vi "compileRfOutputList.vi"(8 "error in (no error)":errorcluster, 11 "ScriptListCompiler in":refnum<class "ScriptListCompiler.lvclass">) -> (0 "error out":errorcluster, 3 "ScriptListCompiler out":refnum<class "ScriptListCompiler.lvclass">)   [LabVIEW 2009, in "Compiler.lvlib" / "ScriptListCompiler.lvclass"]
doc: "Compiles the Analog ScriptList.\n i) Applies the calibration.\n ii) Split Analog List by device.\n iii) Produces digital trigger pulses (for each device) making Digital ScriptLists."
uses:
  ScriptListCompiler.lvclass
  ScriptListCompiler.lvclass/ScriptListCompiler.ctl
  Scripting/ScriptingEvent/ScriptEventList/ScriptEventList.lvclass
  DatabaseHelpers/DbConnection/DeviceDataBase/deviceDataBase.lvclass
  DatabaseHelpers/Database Objects/DeviceArray/DeviceArray.lvclass
  DatabaseHelpers/Database Objects/device/device.lvclass
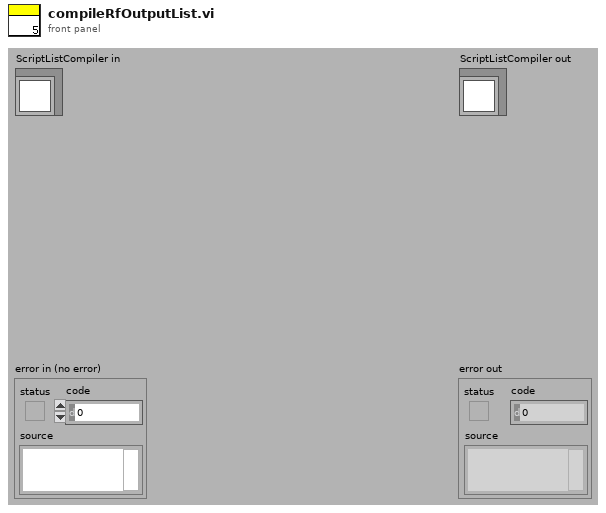
[diagram p1: front panel]
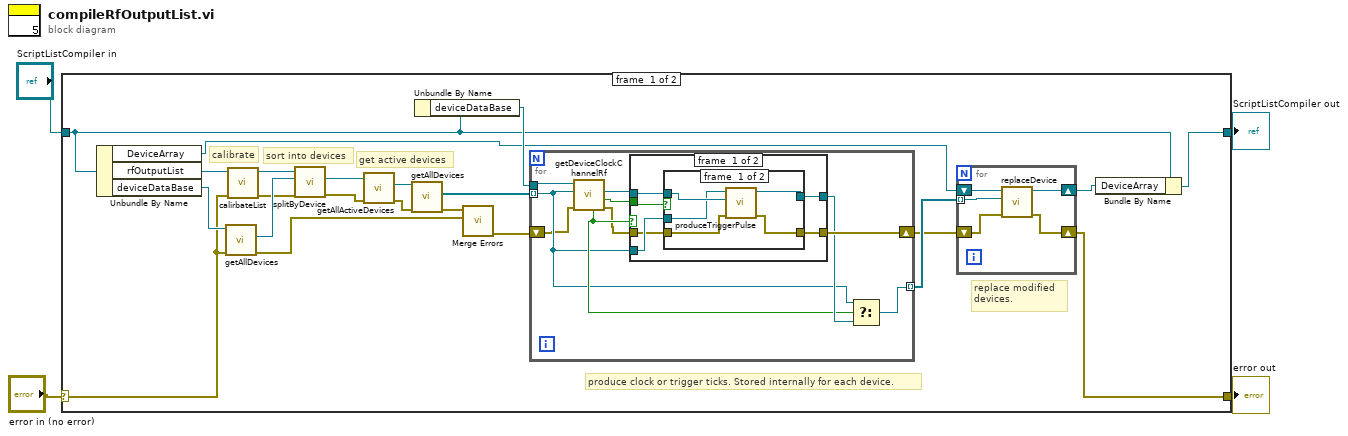
[diagram p0: block diagram]
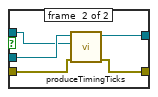
[diagram p2: hidden frame]
diagram:
  n1 = case shown="No Error" "error in (no error)" {
    selector: "error in (no error)" -> [w23 w61]
    tunnel: [w6 w61] -> w3
    tunnel: [w7 w60] -> w1
    tunnel: "ScriptListCompiler in" -> [w8 w60]
    frame #0 {
      # "get active devices"
      # "replace modified \ndevices."
      # "produce clock or trigger ticks. Stored internally for each device."
      # "sort into devices"
      # "calibrate"
      n2 = Unbundle By Name(w8) -> ("DeviceArray"=w5:refnum<class "DeviceArray.lvclass">, "rfOutputList"=w26:refnum<class "ScriptEventList.lvclass">, "deviceDataBase"=w24:refnum<class "deviceDataBase.lvclass">)
      n3 = call "getAllDevices.vi"("error in (no error)"=w23, "deviceDataBase in"=w24) -> ("error out"=w15:errorcluster, "deviceArray.lvclass"=w22:refnum<class "DeviceArray.lvclass">)  [unwired: 7 in, 1 out]
      n4 = call "calirbateList.vi"("error in (no error)"=w23, "ScriptEventList in"=w26) -> ("error out"=w21:errorcluster, "ScriptEventList out"=w25:refnum<class "ScriptEventList.lvclass">)  [unwired: 8 in]
      n5 = call "splitByDevice.vi"("error in (no error)"=w21, "DeviceArray"=w22, "ScriptEventList in"=w25) -> ("error out"=w19:errorcluster, "DeviceArray out"=w20:refnum<class "DeviceArray.lvclass">)  [unwired: 6 in, 1 out]
      n6 = call "getAllActiveDevices.vi"("error in (no error)"=w19, "DeviceArray in"=w20) -> ("error out"=w17:errorcluster, "DeviceArray"=w18:refnum<class "DeviceArray.lvclass">)  [unwired: 7 in, 1 out]
      n7 = call "getAllDevices.vi"("error in (no error)"=w17, "DeviceArray.lvclass in"=w18) -> ("error out"=w16:errorcluster, "deviceArray"=w13:refnum<class "device.lvclass">[])  [unwired: 7 in, 1 out]
      n8 = Unbundle By Name(w8) -> ("deviceDataBase"=w12:refnum<class "deviceDataBase.lvclass">)
      n9 = call <vilib>:"Merge Errors.vi"("error in 2 (no error)"=w15, "error in 1 (no error)"=w16) -> ("error out"=w14:errorcluster)  [unwired: 5 in]
      n10 = for {
        tunnel: w13 -> [w34] mode=indexing
        shift-right: [w41] -> w10
        shift-left: w14 -> [w32]
        tunnel: w12 -> [w35]
        tunnel: [w39] -> w11 mode=indexing
        n11 = call "getDeviceClockChannelRf.vi"("error in (no error)"=w32, "device"=w34, "deviceDataBase in"=w35) -> ("error out"=w33:errorcluster, "isClock"=w37:bool, "timingChannel"=w36:refnum<class "Channel.lvclass">, "noChannel"=w38:bool)  [unwired: 4 in, 1 out]
        n12 = case shown="False" w38 {
          tunnel: w37 -> [w47 _]
          tunnel: w36 -> [w46 _]
          tunnel: w34 -> [w45 w58]
          tunnel: w33 -> [w42 w59]
          tunnel: [w44 w59] -> w41
          tunnel: [w43 w58] -> w40
          frame #0 {
            n13 = case shown="True" w47 {
              tunnel: w46 -> [w51 w56]
              tunnel: w45 -> [w50 w57]
              tunnel: w42 -> [w49 w55]
              tunnel: [w48 w54] -> w44
              tunnel: [w52 w53] -> w43
              frame #0 {
                n14 = call "produceTriggerPulse.vi"("error in (no error)"=w49, "Channel"=w51, "device in"=w50) -> ("error out"=w48:errorcluster, "device out"=w52:refnum<class "device.lvclass">)  [unwired: 7 in]
              }
              frame #1 {
                n15 = call "produceTimingTicks.vi"("error in (no error)"=w55, "Channel"=w56, "device in"=w57) -> ("error out"=w54:errorcluster, "device out"=w53:refnum<class "device.lvclass">)  [unwired: 7 in]
              }
            }
          }
          frame #1 {
          }
        }
        n16 = Select(t=w34, s=w38, f=w40) -> (s? t:f=w39:refnum<class "device.lvclass">)
      }
      n17 = for {
        shift-right: [w27] -> w9
        shift-left: w5 -> [w31]
        tunnel: w11 -> [w30] mode=indexing
        shift-right: [w28] -> w6
        shift-left: w10 -> [w29]
        n18 = call "replaceDevice.vi"("error in (no error)"=w29, "device"=w30, "DeviceArray in"=w31) -> ("error out"=w28:errorcluster, "DeviceArray out"=w27:refnum<class "DeviceArray.lvclass">)  [unwired: 7 in]
      }
      n19 = Bundle By Name(cluster=w8, "DeviceArray"=w9) -> (w7:refnum<class "ScriptListCompiler.lvclass">)
    }
    frame #1 {
    }
  }
  "error out" <- w3
  "ScriptListCompiler out" <- w1
